vi "InitialiseChannelsAngle.vi"(0 "Number of data bits":i32, 5 "Fs":dbl, 11 "error in":errorcluster) -> (4 "output cluster":T1, 15 "error out":errorcluster)   [LabVIEW 2021]
uses:
  <vilib>/DAQmx/create/channels.llb/DAQmx Create Channel (DI-Digital Input).vi
  <vilib>/DAQmx/configure/timing.llb/DAQmx Timing (Sample Clock).vi
  <vilib>/DAQmx/create/channels.llb/DAQmx Create Channel (CO-Pulse Generation-Time).vi
  <vilib>/DAQmx/configure/timing.llb/DAQmx Timing (Implicit).vi
  <vilib>/DAQmx/configure/trigger.llb/DAQmx Start Trigger (Digital Edge).vi
  <vilib>/DAQmx/create/channels.llb/DAQmx Create Channel (CO-Pulse Generation-Frequency).vi
  <resource>/objmgr/daqmx.rc
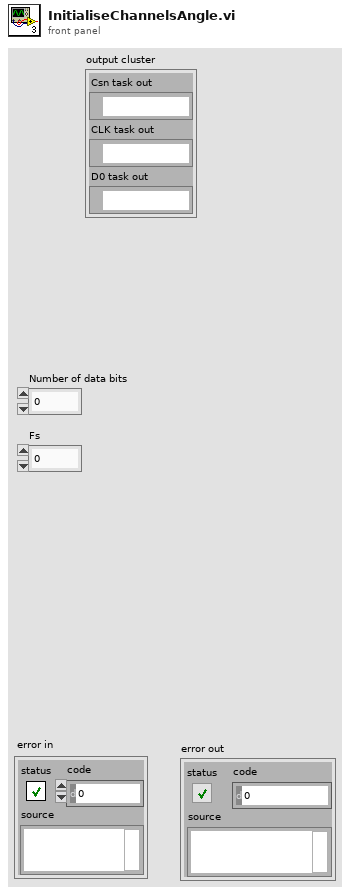
[diagram p1: front panel]
types:
  T1 = cluster{"Csn task out":refnum<k21>, "CLK task out":refnum<k21>, "D0 task out":refnum<k21>}
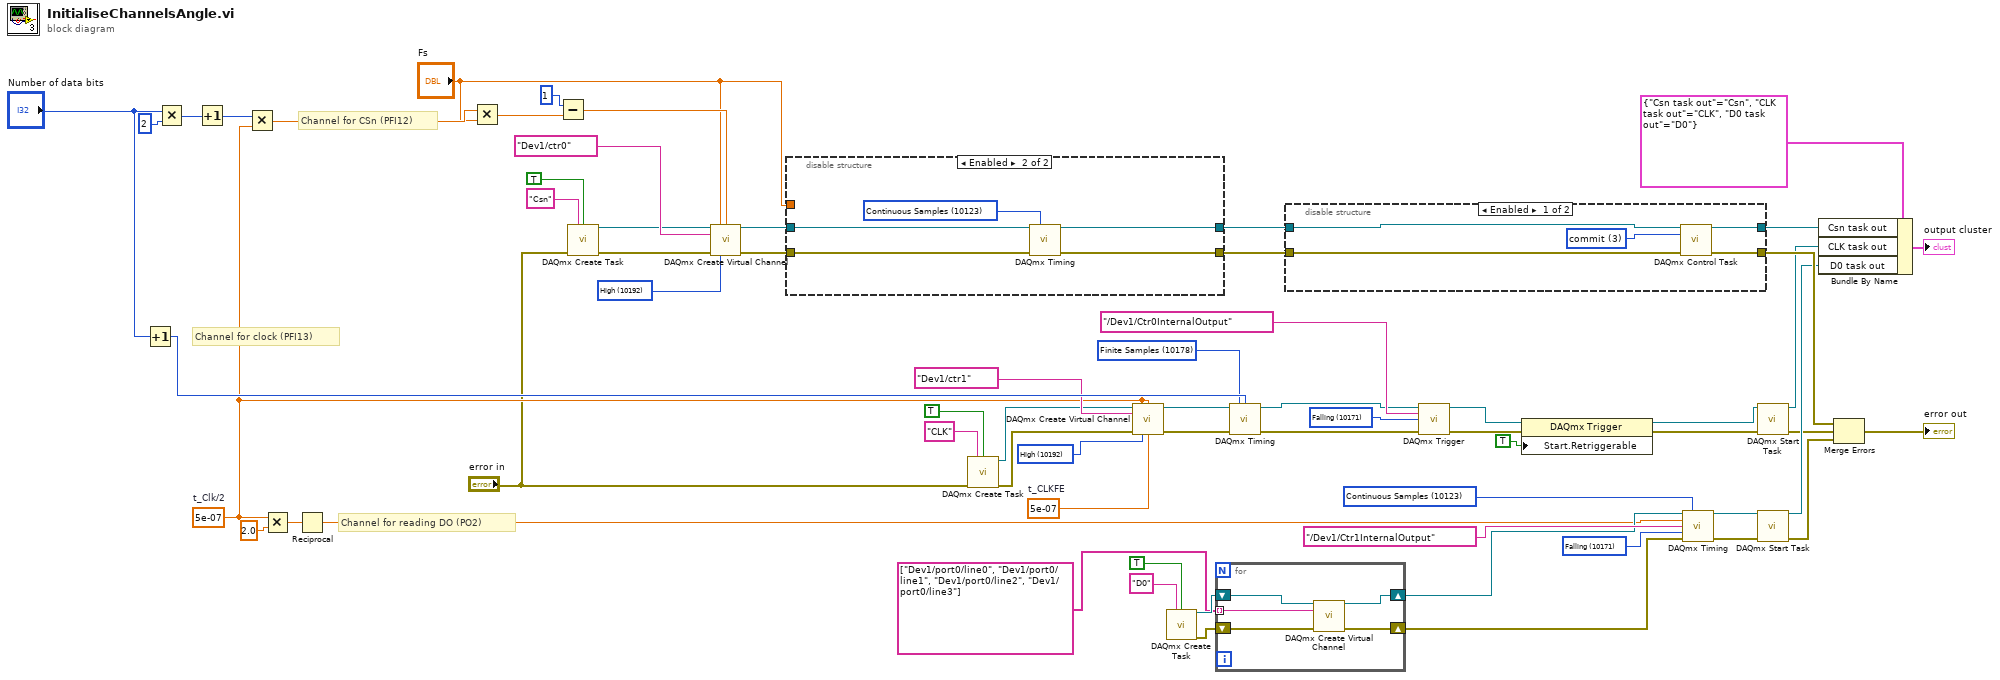
[diagram p0: block diagram]
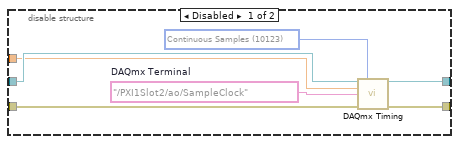
[diagram p2: hidden frame]
diagram:
  w59 = 10192 items=["High"=10192, "Low"=10214] ("idle state")
  w57 = 5e-07  # t_CLKFE
  w46 = 10171 items=["Rising"=10280, "Falling"=10171] ("edge")
  w40 = 10178 items=["Finite Samples"=10178, "Continuous Samples"=10123, "Hardware Timed Single Point"=12522] ("sample mode")
  w38 = 10192 items=["High"=10192, "Low"=10214] ("idle state")
  w16 = 5e-07  # t_Clk/2
  w33 = 10171 items=["Rising"=10280, "Falling"=10171] ("active edge")
  w32 = 10123 items=["Finite Samples"=10178, "Continuous Samples"=10123, "Hardware Timed Single Point"=12522] ("sample mode")
  # "Channel for clock (PFI13)"
  # "Channel for CSn (PFI12)"
  # "Channel for reading DO (PO2)"
  n1 = Increment(x="Number of data bits") -> (x+1=w58:i32)
  n2 = Multiply(x="Number of data bits", y=2) -> (x*y=w35:i32)
  n3 = Increment(x=w35) -> (x+1=w36:i32)
  n4 = Multiply(x=w36, y=w16) -> (x*y=w37:dbl)
  n5 = Multiply(x=w16, y=2.0) -> (x*y=w55:dbl)
  n6 = Reciprocal(x=w55) -> (1/x=w15:dbl)
  n7 = Multiply(x=w37, y="Fs") -> (x*y=w63:dbl)
  n8 = Subtract(x=1, y=w63) -> (x-y=w62:dbl)
  n9 = call <vilib>:"DAQmx Create Task.vi"("new task name"="Csn", "auto cleanup"=TRUE, "error in"="error in") -> ("task out"=w14:refnum<k21>, "error out"=w24:errorcluster)  [unwired: 11 in]
  n10 = call-poly <vilib>:"DAQmx Create Virtual Channel.vi"("task in"=w14, "frequency"="Fs", "duty cycle"=w62, "counter"=tag "Dev1/ctr0", "error in"=w24, "idle state"=w59) -> ("task out"=w52:refnum<k21>, "error out"=w53:errorcluster)  [unwired: 8 in]
  n11 = disable-structure shown="Enabled" {
    disable-tunnel: [w72 w77] -> w54
    disable-tunnel: w53 -> [w71 w76]
    disable-tunnel: w52 -> [w70 w75]
    disable-tunnel: [w69 w74] -> w51
    disable-tunnel: "Fs" -> [w66 _]
    frame Disabled {
      w67 = tag "/PXI1Slot2/ao/SampleClock"  # DAQmx Terminal
      w68 = 10123 items=["Finite Samples"=10178, "Continuous Samples"=10123, "Hardware Timed Single Point"=12522] ("sample mode")
      n12 = call-poly <vilib>:"DAQmx Timing.vi"("task/channels in"=w70, "sample mode"=w68, "rate"=w66, "source"=w67, "error in"=w71) -> ("task out"=w69:refnum<k21>, "error out"=w72:errorcluster)  [unwired: 9 in]
    }
    frame Enabled {
      w73 = 10123 items=["Finite Samples"=10178, "Continuous Samples"=10123, "Hardware Timed Single Point"=12522] ("sample mode")
      n13 = call-poly <vilib>:"DAQmx Timing.vi"("task/channels in"=w75, "sample mode"=w73, "error in"=w76) -> ("task out"=w74:refnum<k21>, "error out"=w77:errorcluster)  [unwired: 11 in]
    }
  }
  n14 = call <vilib>:"DAQmx Create Task.vi"("new task name"="CLK", "auto cleanup"=TRUE, "error in"="error in") -> ("task out"=w20:refnum<k21>, "error out"=w21:errorcluster)  [unwired: 11 in]
  n15 = call-poly <vilib>:"DAQmx Create Virtual Channel.vi"("task in"=w20, "high time"=w16, "low time"=w16, "counter"=tag "Dev1/ctr1", "error in"=w21, "idle state"=w38, "initial delay"=w57) -> ("task out"=w41:refnum<k21>, "error out"=w42:errorcluster)  [unwired: 7 in]
  n16 = call <vilib>:"DAQmx Create Task.vi"("new task name"="D0", "auto cleanup"=TRUE) -> ("task out"=w31:refnum<k21>, "error out"=w30:errorcluster)  [unwired: 12 in]
  n17 = for {
    tunnel: tag[] ["Dev1/port0/line0", "Dev1/port0/line1", "Dev1/port0/line2", "Dev1/port0/line3"] ("DAQmx Output Channels") -> [w80] mode=indexing
    shift-right: [w79] -> w28
    shift-left: w31 -> [w82]
    shift-right: [w78] -> w27
    shift-left: w30 -> [w81]
    n18 = call-poly <vilib>:"DAQmx Create Virtual Channel.vi"("task in"=w82, "lines"=w80, "error in"=w81) -> ("task out"=w79:refnum<k21>, "error out"=w78:errorcluster)  [unwired: 11 in]
  }
  n19 = call-poly <vilib>:"DAQmx Timing.vi"("task/channels in"=w41, "sample mode"=w40, "samples per channel"=w58, "error in"=w42) -> ("task out"=w43:refnum<k21>, "error out"=w44:errorcluster)  [unwired: 10 in]
  n20 = disable-structure shown="Enabled" {
    disable-tunnel: [w87 w88] -> w25
    disable-tunnel: w51 -> [w85 w89]
    disable-tunnel: w54 -> [w84 w88]
    disable-tunnel: [w83 w89] -> w12
    frame Enabled {
      w86 = 3 items=["verify"=2, "reserve"=4, "commit"=3, "unreserve"=5, "abort"=6] ("action")
      n21 = call <vilib>:"DAQmx Control Task.vi"("task/channels in"=w85, "action"=w86, "error in"=w84) -> ("task out"=w83:refnum<k21>, "error out"=w87:errorcluster)  [unwired: 11 in]
    }
    frame Disabled {
    }
  }
  n22 = call-poly <vilib>:"DAQmx Trigger.vi"("task/channels in"=w43, "source"=tag "/Dev1/Ctr0InternalOutput", "edge"=w46, "error in"=w44) -> ("task out"=w47:refnum<k21>, "error out"=w49:errorcluster)  [unwired: 10 in]
  n23 = property class="DAQmx Trigger"(reference=w47, error in=w49, "Start.Retriggerable"=TRUE) -> (reference out=w11:refnum<k21>, error out=w6:errorcluster)
  n24 = call-poly <vilib>:"DAQmx Timing.vi"("task/channels in"=w28, "sample mode"=w32, "rate"=w15, "source"=tag "/Dev1/Ctr1InternalOutput", "active edge"=w33, "error in"=w27) -> ("task out"=w9:refnum<k21>, "error out"=w5:errorcluster)  [unwired: 8 in]
  n25 = call <vilib>:"DAQmx Start Task.vi"("task/channels in"=w11, "error in"=w6) -> ("task out"=w10:refnum<k21>, "error out"=w7:errorcluster)  [unwired: 12 in]
  n26 = call <vilib>:"DAQmx Start Task.vi"("task/channels in"=w9, "error in"=w5) -> ("task out"=w8:refnum<k21>, "error out"=w4:errorcluster)  [unwired: 12 in]
  n27 = Bundle By Name(cluster=T1 {"Csn task out"="Csn", "CLK task out"="CLK", "D0 task out"="D0"}, "Csn task out"=w12, "CLK task out"=w10, "D0 task out"=w8) -> (→"output cluster":T1)
  n28 = Merge Errors(w25, w7, w4) -> (→"error out":errorcluster)
